vi "Temperature.vi"(0 "second channel":i8, 2 "selected calibration array":T1 {"D.O."."K" format="%.6f"; "D.O."."Temperature" format="%.2f"; "pH scale"."Buffers"."V/T" format="%.5f"; "pH scale"."Buffers"."Buffer" format="%.2f"; "pH scale"."Temperature" format="%.2f"; "offset (physical units)" format="%.5f"; "correspondence table"."volts" format="%.4f"; "correspondence table"."physical units" format="%.4f"; "second channel" min=-1; "offset (volts)" format="%.5f"; "conversion matrix" format="%.4e"}, 3 "voltage data":sgl[](array[numeric]) format="%.2f", 4 "Default Temperature (C)":dbl=20.0 format="%.2f") -> (5 "Temperature (C)":dbl format="%.2f")   [LabVIEW 2015]
uses:
  calib array.ctl
  conversion.ctl
  DAQ configuration/scale type.ctl
  correspondence table.ctl
  pH/pH scale.ctl
  Dissolved Oxygen/DO scale.ctl
  Spectrophotometer/Photometer calibration data.ctl
panel:
  # "C"
  # "kPa"
  # "C"
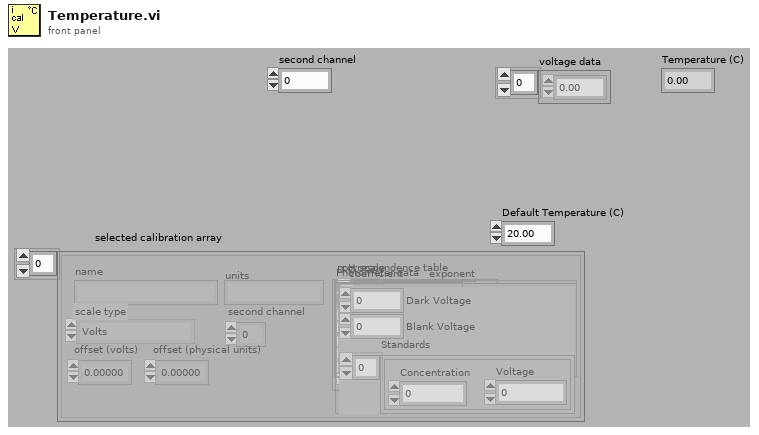
[diagram p1: front panel]
types:
  T1 = typedef "calib array.ctl" = T2[]
  T2 = typedef "conversion.ctl" = cluster{"conversion matrix":sgl[][], "units":string, "name":string, "scale type":T3, "offset (volts)":dbl, "second channel":i8, "correspondence table":T4, "offset (physical units)":dbl, "pH scale":T5, "D.O.":T6, "Photometer data":T7}
  T3 = typedef "scale type.ctl" = enum16{"Volts", "Polynomial", "Correspondence Table", "pH", "Dissolved Oxygen", "Quadratic", "Photometer"}
  T4 = typedef "correspondence table.ctl" = cluster{"physical units":dbl, "volts":dbl}[]
  T5 = typedef "pH scale.ctl" = cluster{"Buffers":cluster{"Buffer":dbl, "Calibrated":bool, "V/T":dbl}[], "Temperature":dbl}
  T6 = typedef "DO scale.ctl" = cluster{"Temperature":dbl, "K":dbl, "barometric pressure":dbl}
  T7 = typedef "Photometer calibration data.ctl" = cluster{"Dark Voltage":dbl, "Blank Voltage":dbl, "Standards":cluster{"Concentration":dbl, "Voltage":dbl}[]}
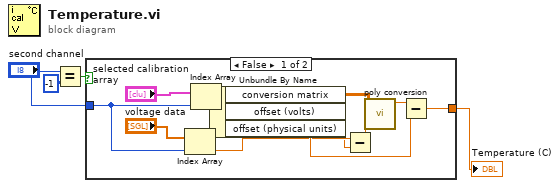
[diagram p0: block diagram]
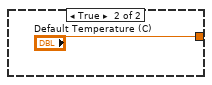
[diagram p2: hidden frame]
diagram:
  n1 = Equal?(x="second channel", y=i8 -1) -> (x = y?=w1:bool)
  n2 = case shown="False" w1 {
    tunnel: "second channel" -> [w5 _]
    tunnel: [w14 "Default Temperature (C)"] -> w2
    frame False {
      n3 = Index Array(array="voltage data", index=w5) -> (element=w11:sgl)
      n4 = Index Array(array="selected calibration array", index=w5) -> (element=w7:T2)
      n5 = Unbundle By Name(w7) -> ("conversion matrix"=w8:sgl[][], "offset (volts)"=w10:dbl, "offset (physical units)"=w15:dbl)
      n6 = Subtract(x=w11, y=w10) -> (x-y=w12:dbl)
      n7 = call "poly conversion.vi"("Volts"=w12, "conversion matrix"=w8) -> ("Calibrated value"=w13:dbl)  [unwired: 9 in]
      n8 = Subtract(x=w13, y=w15) -> (x-y=w14:dbl)
    }
    frame True {
    }
  }
  "Temperature (C)" <- w2
